vi "Ex2Camerascascadeorcoolsnap.vi"() -> ()   [LabVIEW 2010]
panel:
  in  "overlap mode 2":bool
  in  "overlap mode 1":bool
  in  "camera 2 name":string
  in  "camera 1 name":string
  in  "Store 2":bool
  in  "stop 2":bool
  in  "Store":bool
  in  "stop":bool
  in  "Intensifier Camera 2":bool
  in  "Intensifier Camera 1":bool
  in  "Exposure Camera 2":dbl=0.5 format="%.2f"
  in  "Exposure Camera 1":dbl=0.5 format="%.2f"
  out "error out":errorcluster
  in  "error in (no error)":errorcluster
  # "Ex2Cameras:\nThis example runs two cameras in focus mode. Remember to setup two cameras in the pvcam.ini file. This example is setup for the Cascade, PhotonMax, and CoolSnap. For the \nCascade and PhotonMax the user may want to add the shift register and avalanche gain."
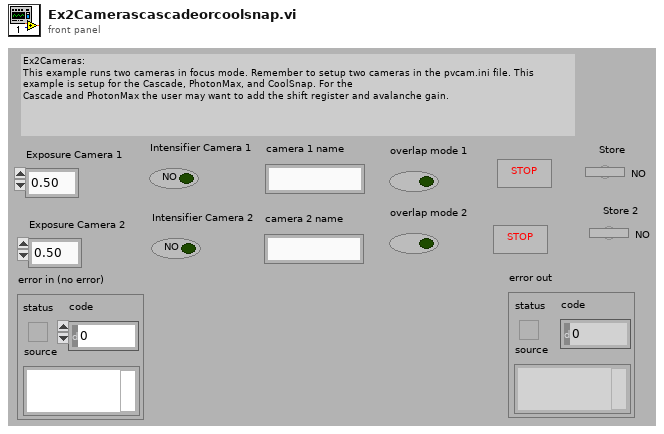
[diagram p1: front panel]
types:
  T1 = cluster{"Camera Handle":u32, "Pulser Handle":u32, "File Handle":u32, "Display Handle":u32, "Image Handle":u32}
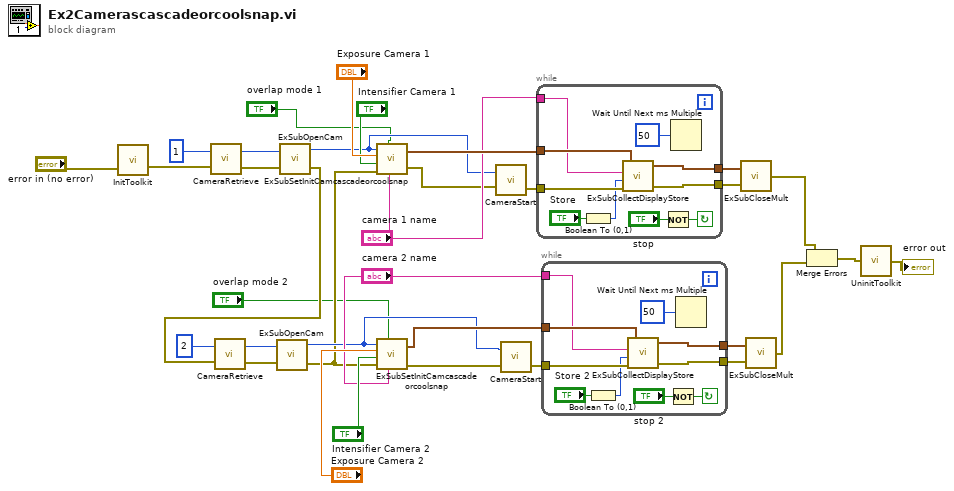
[diagram p0: block diagram]
diagram:
  n1 = call <userlib>:"InitToolkit.vi"("error in"="error in (no error)") -> ("error out"=w8:errorcluster)
  n2 = call <userlib>:"CameraRetrieve.vi"("error in"=w8, "Camera Index"=1) -> ("error out"=w10:errorcluster, "Device ID"=w9:u32)
  n3 = call "ExSubOpenCam.vi"("error in (no error)"=w10, "Camera Device ID"=w9) -> ("error out"=w4:errorcluster, "Camera Handle"=w20:u32)
  n4 = call <userlib>:"CameraRetrieve.vi"("error in"=w4, "Camera Index"=2) -> ("error out"=w5:errorcluster, "Device ID"=w6:u32)
  n5 = call "ExSubOpenCam.vi"("error in (no error)"=w5, "Camera Device ID"=w6) -> ("error out"=w11:errorcluster, "Camera Handle"=w19:u32)
  n6 = call "ExSubSetInitCamcascadeorcoolsnap.vi"("Name"="camera 1 name", "overlap mode"="overlap mode 1", "error in (no error)"=w11, "Intensifier"="Intensifier Camera 1", "Exposure"="Exposure Camera 1", "Camera Handle"=w20) -> ("error out"=w14:errorcluster, "Handles Out"=w23:T1)
  n7 = call "ExSubSetInitCamcascadeorcoolsnap.vi"("Name"="camera 2 name", "overlap mode"="overlap mode 2", "error in (no error)"=w11, "Intensifier"="Intensifier Camera 2", "Exposure"="Exposure Camera 2", "Camera Handle"=w19) -> ("error out"=w13:errorcluster, "Handles Out"=w24:T1)
  n8 = call <userlib>:"CameraStart.vi"("error in"=w14, "Camera Handle"=w20) -> ("error out"=w12:errorcluster)  [unwired: 1 out]
  n9 = call <userlib>:"CameraStart.vi"("error in"=w13, "Camera Handle"=w19) -> ("error out"=w25:errorcluster)  [unwired: 1 out]
  n10 = while {
    tunnel: w23 -> [w43]
    tunnel: w12 -> [w42]
    tunnel: "camera 1 name" -> [w35]
    tunnel: [w40] -> w28
    tunnel: [w41] -> w29
    stop <- w38 continue-if-true
    n11 = Boolean To (0,1)(Boolean="Store") -> (0, 1=w36:i16)
    n12 = call "ExSubCollectDisplayStore.vi"("error in (no error)"=w42, "Store flag"=w36, "Display Title"=w35, "Handle Cluster"=w43) -> ("error out"=w40:errorcluster, "Handle Cluster Out"=w41:T1)  [unwired: 1 out]
    n13 = Not(x="stop") -> (.not. x?=w38:bool)
    n14 = Wait Until Next ms Multiple(millisecond multiple=u32 50) -> ()  [unwired: 1 out]
  }
  n15 = while {
    tunnel: w24 -> [w53]
    tunnel: w25 -> [w52]
    tunnel: "camera 2 name" -> [w45]
    tunnel: [w50] -> w26
    tunnel: [w51] -> w27
    stop <- w48 continue-if-true
    n16 = Boolean To (0,1)(Boolean="Store 2") -> (0, 1=w46:i16)
    n17 = call "ExSubCollectDisplayStore.vi"("error in (no error)"=w52, "Store flag"=w46, "Display Title"=w45, "Handle Cluster"=w53) -> ("error out"=w50:errorcluster, "Handle Cluster Out"=w51:T1)  [unwired: 1 out]
    n18 = Not(x="stop 2") -> (.not. x?=w48:bool)
    n19 = Wait Until Next ms Multiple(millisecond multiple=u32 50) -> ()  [unwired: 1 out]
  }
  n20 = call "ExSubCloseMult.vi"("error in (no error)"=w28, "Handles In"=w29) -> ("error out"=w16:errorcluster)
  n21 = call "ExSubCloseMult.vi"("error in (no error)"=w26, "Handles In"=w27) -> ("error out"=w15:errorcluster)
  n22 = Merge Errors(w16, w15) -> (w18:errorcluster)
  n23 = call <userlib>:"UninitToolkit.vi"("error in"=w18) -> ("error out"=→"error out":errorcluster)
